vi "Derivativa.vi"(1 "Kd":dbl, 2 "Dt":dbl, 3 "Valor Anterior":dbl) -> (0 "Acción derivativa":dbl)   [LabVIEW 2011]
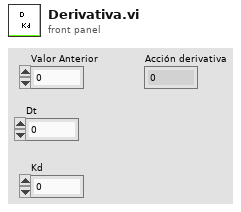
[diagram p1: front panel]
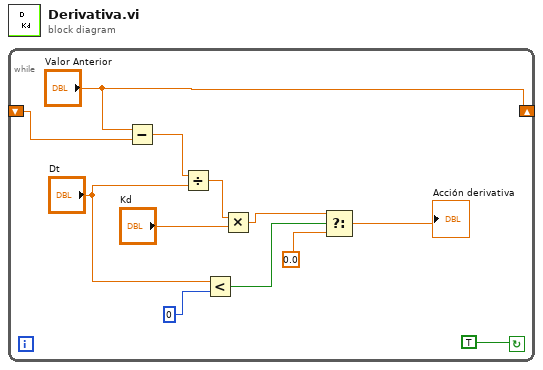
[diagram p0: block diagram]
diagram:
  n1 = while {
    shift-right: ["Valor Anterior"] -> _
    shift-left: _ -> [w10]
    stop <- TRUE continue-if-true
    n2 = Subtract(x="Valor Anterior", y=w10) -> (x-y=w9:dbl)
    n3 = Divide(x=w9, y="Dt") -> (x/y=w8:dbl)
    n4 = Less?(x="Dt", y=0) -> (x < y?=w4:bool)
    n5 = Multiply(x=w8, y="Kd") -> (x*y=w3:dbl)
    n6 = Select(t=w3, s=w4, f=0.0) -> (s? t:f=→"Acción derivativa":dbl)
  }
